vi "Memory.Pointer.Write.Safe.1D.U8.vi"(8 "error in (no error)":errorcluster, 9 "count":u64 format="%d elements", 10 "buffer in":u8[](array[numeric]), 11 "pointer in":refnum<class "Memory.Pointer.lvclass">) -> (0 "error out":errorcluster, 2 "buffer out":u8[](array[numeric]), 3 "pointer out":refnum<class "Memory.Pointer.lvclass">)   [LabVIEW 2016, in "Memory Manager.lvlib" / "Memory.Pointer.lvclass"]
doc: "Writes <b>count</b> elements from the provided <b>buffer</b> to the address specified by <b>pointer</b>.\n\n<b>Note:</b> This VI is <b>unsafe</b>.\n\nUnsafe means that it does not evaluate the size parameter of <b>pointer</b> to ensure that is inbounds of allocated memory before peforming a memory read/write. Reading/writing more data to a pointer than it has allocated can corrupt or crash LabVIEW. Only use this VI in scenarios where the <b>pointer</b> has been validated to be allocated to a correct size before calling this VI."
uses:
  Memory.Pointer.lvclass
  Memory.Pointer.lvclass/Memory.Pointer.ctl
  Accessors/Get Address.vi
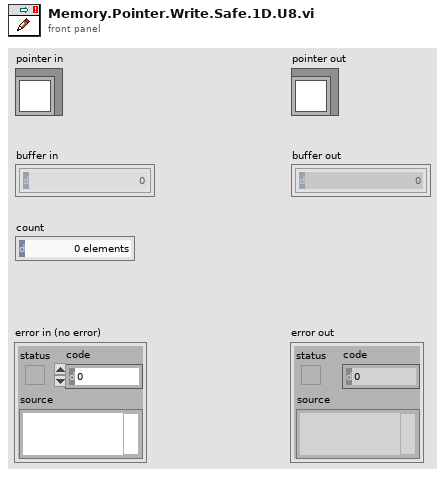
[diagram p1: front panel]
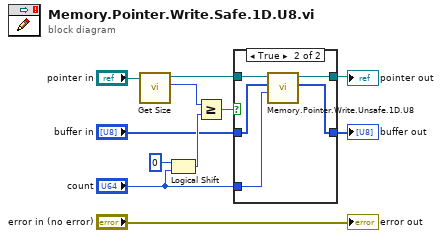
[diagram p0: block diagram]
diagram:
  n1 = call "Get Size.vi"("Pointer in"="pointer in") -> ("size"=w9:u64, "Pointer out"=w6:refnum<class "Memory.Pointer.lvclass">)  [unwired: 8 in, 1 out]
  n2 = Logical Shift(y=i16 0, x="count") -> (x << y=w8:u64)
  n3 = Greater Or Equal?(x=w9, y=w8) -> (x >= y?=w7:bool)
  n4 = case shown="True" w7 {
    tunnel: w6 -> [w13 w18]
    tunnel: [w13 w17] -> w5
    tunnel: "buffer in" -> [w12 w16]
    tunnel: "count" -> [_ w15]
    tunnel: [w12 w14] -> w2
    frame False {
    }
    frame True {
      n5 = call "Memory.Pointer.Write.Unsafe.1D.U8.vi"("count"=w15, "buffer in"=w16, "pointer in"=w18) -> ("buffer out"=w14:u8[], "pointer out"=w17:refnum<class "Memory.Pointer.lvclass">)  [unwired: 6 in, 1 out]
    }
  }
  "pointer out" <- w5
  "buffer out" <- w2
  "error out" <- "error in (no error)"
